vi "定位状态.vi"(8 "error in (no error)":errorcluster) -> (0 "error out":errorcluster, 3 "状态":u16(ring) items=["待机", "定位中", "定位完成"])   [LabVIEW 2016, in "PLC.lvlib"]
uses:
  PLC.lvlib
  <vilib>/Plasmionique/MB Master/MB_Master_Serial/MB_Master_Serial.lvclass
  C:/Program Files (x86)/National Instruments/LabVIEW 2016/vi.lib/Plasmionique/MB Master/MB_Master/MB_Master.lvclass
  <vilib>/Plasmionique/MB Master/MB Master.lvlib
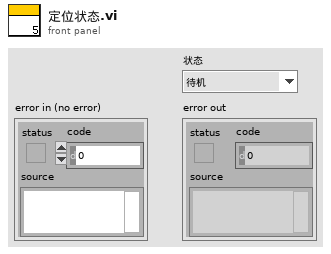
[diagram p1: front panel]
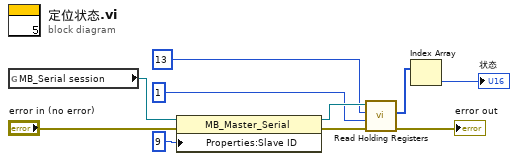
[diagram p0: block diagram]
diagram:
  n1 = global read "中间变量.vi" "MB_Serial session"() -> (w9:refnum<class "MB_Master_Serial.lvclass">)
  n2 = property class="MB_Master_Serial"(reference=w9, error in="error in (no error)", "Properties:Slave ID"=u8 9 ("Slave ID")) -> (reference out=w8:refnum<class "MB_Master_Serial.lvclass">, error out=w5:errorcluster)
  n3 = call <vilib>:"Read Holding Registers.vi"("error in (no error)"=w5, "quantity"=u16 1, "starting address"=u16 13, "MB session in"=w8) -> ("error out"=→"error out":errorcluster, "Registers"=w2:u16[])  [unwired: 5 in, 1 out]
  n4 = Index Array(array=w2) -> (element=→"状态":u16)  [unwired: 1 in]
